vi "log.vi"(11 "log":string) -> ()   [LabVIEW 2022 SP3, in "工况数据上传.lvlib"]
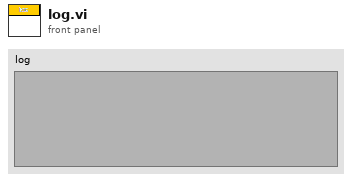
[diagram p1: front panel]
types:
  T1 = enum16{"open", "replace", "create", "open or create", "replace or create", "replace or create with confirmation"}
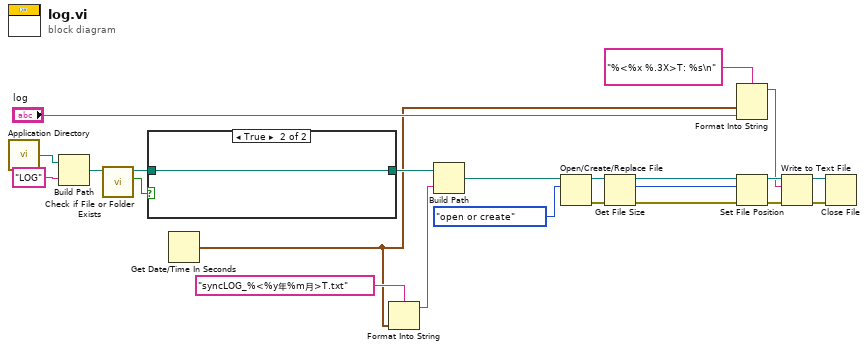
[diagram p0: block diagram]
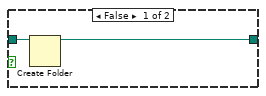
[diagram p2: hidden frame]
diagram:
  n1 = call <vilib>:"Application Directory.vi"() -> ("Application Directory"=w23:path)
  n2 = Build Path(base path=w23, name or relative path="LOG" ("名称或相对路径")) -> (appended path=w10:path)
  n3 = call <vilib>:"Check if File or Folder Exists.vi"("path"=w10) -> ("file or folder exists?"=w9:bool, "dup path"=w8:path)  [unwired: 8 in, 1 out]
  n4 = case shown="True" w9 {
    tunnel: w8 -> [w25 w26]
    tunnel: [w24 w26] -> w7
    frame False {
      n5 = Create Folder(path (use dialog)=w25) -> (created path=w24:path)  [unwired: 2 in, 2 out]
    }
    frame True {
    }
  }
  n6 = Get Date/Time In Seconds() -> (seconds since 1Jan1904=w3:timestamp)
  n7 = Format Into String(format string="syncLOG_%<%y年%m月>T.txt" ("格式字符串"), w3) -> (resulting string=w2:string)  [unwired: 2 in, 1 out]
  n8 = Build Path(base path=w7, name or relative path=w2) -> (appended path=w21:path)
  n9 = Open/Create/Replace File(file path (use dialog)=w21, operation (0:open)=T1."open or create" ("操作(0:open)")) -> (refnum out=w5:refnum<file>, error out=w16:errorcluster)  [unwired: 4 in, 1 out]
  n10 = Get File Size(file=w5, error in=w16) -> (refnum out=w19:refnum<file>, size (in bytes)=w6:i64, 0:w18:errorcluster)
  n11 = Format Into String(format string="%<%x %.3X>T: %s\n" ("格式字符串"), w3, "log") -> (resulting string=w11:string)  [unwired: 2 in, 1 out]
  n12 = Set File Position(offset (in bytes) (0)=w6, refnum=w19, error in=w18) -> (refnum out=w17:refnum<file>, error out=w15:errorcluster)  [unwired: 1 in]
  n13 = Write to Text File(file (use dialog)=w17, text=w11, error in=w15) -> (refnum out=w1:refnum<file>, error out=w14:errorcluster)  [unwired: 1 in, 1 out]
  n14 = Close File(refnum=w1, error in=w14) -> ()  [unwired: 2 out]
